vi "data_to_xml.vi"(8 "error in (no error)":errorcluster, 11 "Experiment in":refnum<class "Experiment.lvclass">) -> (0 "error out":errorcluster, 2 "data string":string, 3 "Experiment out":refnum<class "Experiment.lvclass">)   [LabVIEW 2013, in "Experiment.lvclass"]
uses:
  Experiment.lvclass
  Experiment.lvclass/Experiment.ctl
  Camera/Hamamatsu_C9100-13/Hamamatsu_C9100-13.lvclass
  Counter/Counter.lvclass
  TTL_input/TTL_input.lvclass
  Globals.vi
  Camera/Camera.lvclass
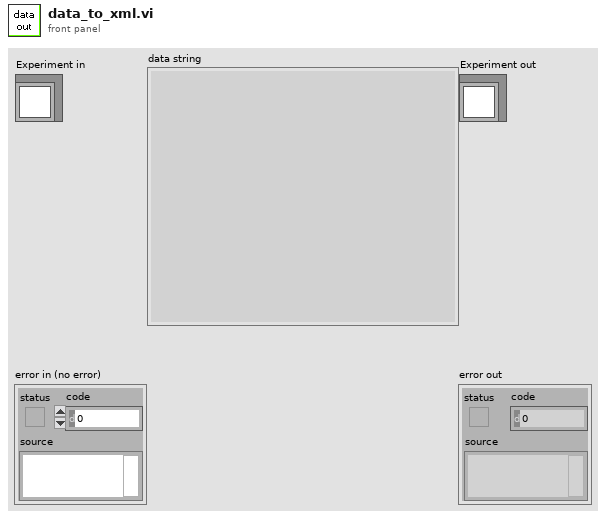
[diagram p1: front panel]
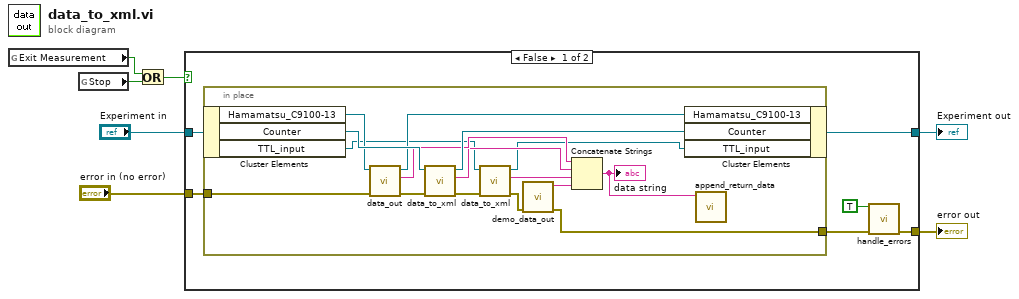
[diagram p0: block diagram]
diagram:
  n1 = global read "Globals.vi" "Exit Measurement"() -> (w4:bool)
  n2 = global read "Globals.vi" "Stop"() -> (w3:bool)
  n3 = Or(x=w4, y=w3) -> (x .or. y?=w2:bool)
  n4 = case shown="False" w2 {
    tunnel: [w12 w31] -> w6
    tunnel: "Experiment in" -> [w13 w31]
    tunnel: [w10 w30] -> w5
    tunnel: "error in (no error)" -> [w8 w30]
    frame False {
      n5 = in-place {
        in-place-border: [w16] -> w11
        in-place-border: w8 -> [w24]
        n6 = in-place-cluster #1(w13) -> ("Hamamatsu_C9100-13"=w27:refnum<class "Hamamatsu_C9100-13.lvclass">, "Counter"=w29:refnum<class "Counter.lvclass">, "TTL_input"=w21:refnum<class "TTL_input.lvclass">)
        n7 = call-dynamic "data_out.vi"("error in (no error)"=w24, "Hamamatsu_C9100-13 in"=w27) -> ("error out"=w25:errorcluster, "camera data string"=w23:string, "Hamamatsu_C9100-13 out"=w26:refnum<class "Hamamatsu_C9100-13.lvclass">)  [unwired: 7 in]
        n8 = call-dynamic "data_to_xml.vi"("error in (no error)"=w25, "Counter in"=w29) -> ("error out"=w19:errorcluster, "counter data string"=w22:string, "Counter out"=w28:refnum<class "Counter.lvclass">)  [unwired: 7 in]
        n9 = call-dynamic "data_to_xml.vi"("error in (no error)"=w19, "TTL_input in"=w21) -> ("error out"=w17:errorcluster, "TTL data string"=w18:string, "TTL_input out"=w20:refnum<class "TTL_input.lvclass">)  [unwired: 7 in]
        n10 = call "demo_data_out.vi"("error in (no error)"=w17) -> ("error out"=w16:errorcluster, "camera data string"=w15:string)  [unwired: 9 in]
        n11 = Concatenate Strings(w23, w22, w18, w15) -> (w14:string)
        "data string" <- w14
        n12 = in-place-cluster #1("Hamamatsu_C9100-13"=w26, "Counter"=w28, "TTL_input"=w20) -> (w12:refnum<class "Experiment.lvclass">)
        n13 = call "append_return_data.vi"("Return Data"=w14) -> ()  [unwired: 11 in]
      }
      n14 = call "handle_errors.vi"("Exit Operation"=TRUE ("Exit Measurement"), "error in (no error)"=w11) -> ("error out"=w10:errorcluster)  [unwired: 13 in]
    }
    frame True {
    }
  }
  "error out" <- w5
  "Experiment out" <- w6
